vi "Find Msgs.vi"(10 "X Actor.lvclass":variant) -> (2 "Msgs":T1)   [LabVIEW 2025, in "jettl.lvlib"]
uses:
  jettl.lvlib
  Msgs.ctl
  Msg/Msg.lvclass
  <vilib>/Utility/Data Type/NI_Data Type.lvlib
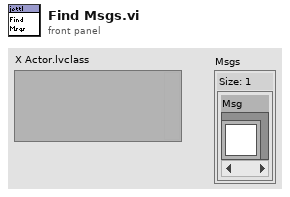
[diagram p1: front panel]
types:
  T1 = typedef "jettl.lvlib/Msgs.ctl" = set{refnum<class "Msg.lvclass">}
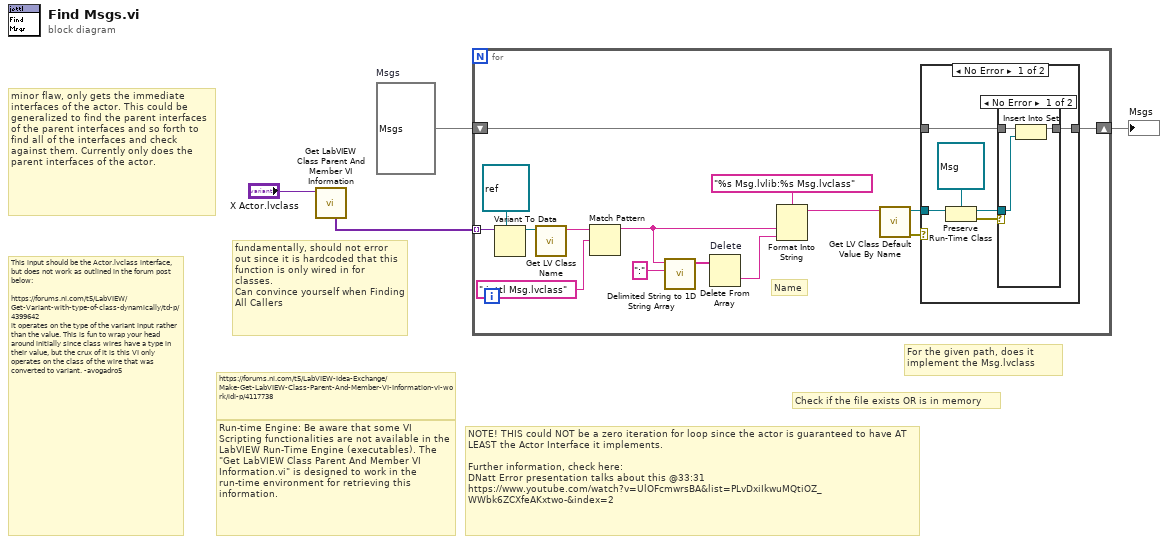
[diagram p0: block diagram]
diagram:
  w3 = T1 {}  # Msgs
  # "fundamentally, should not error out since it is hardcoded that this function is only wired in for classes.\nCan convince yourself when Finding All Callers"
  # "Check if the file exists OR is in memory"
  # "For the given path, does it implement the Msg.lvclass"
  # "NOTE! THIS could NOT be a zero iteration for loop since the actor is guaranteed to have AT LEAST the Actor Interface it implements.\n\nFurther information, check here:\nDNatt Error presentation talks about this @33:31\nhttps://www.youtube.com/watch?v=UlOFcmwrsBA&list=PLvDxiIkwuMQtiOZ_WWbk6ZCXfeAKxtwo-&index=2"
  # "This input should be the Actor.lvclass interface, but does not work as outlined in the forum post below:\n\nhttps://forums.ni.com/t5/LabVIEW/Get-Variant-with-type-of-class-dynamically/td-p/4399642\nit operates on the type of the variant input rather than the value. This is fun to wrap your head around initially since class wires have a type in their value, but the crux of it is this VI only operates on the class of the wire that was converted to variant. -avogadro5"
  # "minor flaw, only gets the immediate interfaces of the actor. This could be generalized to find the parent interfaces of the parent interfaces and so forth to find all of the interfaces and check against them. Currently only does the parent interfaces of the actor."
  # "Run-time Engine: Be aware that some VI Scripting functionalities are not available in the LabVIEW Run-Time Engine (executables). The \"Get LabVIEW Class Parent And Member VI Information.vi\" is designed to work in the run-time environment for retrieving this information."
  # "https://forums.ni.com/t5/LabVIEW-Idea-Exchange/Make-Get-LabVIEW-Class-Parent-And-Member-VI-Information-vi-work/idi-p/4117738"
  n1 = call <vilib>:"Get LabVIEW Class Parent And Member VI Information.vi"("variant"="X Actor.lvclass") -> ("parent interfaces"=w4:variant[])  [unwired: 7 in, 3 out]
  n2 = for {
    tunnel: w4 -> [w18] mode=indexing
    shift-right: [w14] -> w2
    shift-left: w3 -> [w15]
    # "Name"
    n3 = Variant To Data(type=refnum<class> refnum ("LabVIEW Object"), Variant=w18) -> (data=w17:refnum<class>)  [unwired: 1 in, 1 out]
    n4 = call <vilib>:"Get LV Class Name.vi"("object"=w17) -> ("class name"=w13:string)  [unwired: 9 in, 1 out]
    n5 = Match Pattern(string=w13, regular expression=" jettl Msg.lvclass" ("string")) -> (before substring=w7:string)  [unwired: 1 in, 3 out]
    n6 = call <vilib>:"Delimited String to 1D String Array.vi"("delimiter"=":", "delimited string"=w7) -> ("string array"=w6:string[])  [unwired: 9 in]
    n7 = Delete From Array "Delete"(array=w6) -> (deleted portion=w5:string)  [unwired: 2 in, 1 out]
    n8 = Format Into String(format string="%s Msg.lvlib:%s Msg.lvclass", w7, w5) -> (resulting string=w9:string)  [unwired: 2 in, 1 out]
    n9 = call <vilib>:"Get LV Class Default Value By Name.vi"("class name"=w9) -> ("error out"=w11:errorcluster, "object"=w16:refnum<class>)  [unwired: 9 in]
    n10 = case shown="No Error" w11 {
      tunnel: w16 -> [w22 _]
      tunnel: w15 -> [w21 w30]
      tunnel: [w20 w30] -> w14
      frame No Error {
        n11 = Preserve Run-Time Class(object in=w22, 2:refnum<class "Msg.lvclass"> refnum ("Msg")) -> (object out=w25:refnum<class "Msg.lvclass">, error out=w23:errorcluster)  [unwired: 1 in]
        n12 = case shown="No Error" w23 {
          tunnel: w21 -> [w28 w29]
          tunnel: [w27 w29] -> w20
          tunnel: w25 -> [w26 _]
          frame No Error {
            n13 = Insert Into Set(10:w26, 11:w28) -> (3:w27:T1)  [unwired: 1 out]
          }
          frame Error {
          }
        }
      }
      frame Error {
      }
    }
  }
  "Msgs" <- w2
